vi "init_read_test.vi"() -> ()   [LabVIEW 2020, in "Avantes_bunch.lvclass"]
uses:
  Avantes_bunch.lvclass
  C:/dev/TRANCON/Classes/GeneralFunctionality/GeneralFunctionality.lvclass
  Config/config_names_def.ctl
  Config/Config.lvclass
  GeneralFunctionality/GeneralFunctionality.lvclass/GeneralFunctionality.ctl
  GeneralFunctionality/GeneralFunctionality.lvclass
panel:
  out "Waveform Graph 2":sgl[](graph)
  out "Waveform Graph":sgl[](graph)
  out "measuring":i32
  out "error out":errorcluster
  in  "Path":path=path "C:/Dev/TRANCON/settings/settingsDetector.ini"
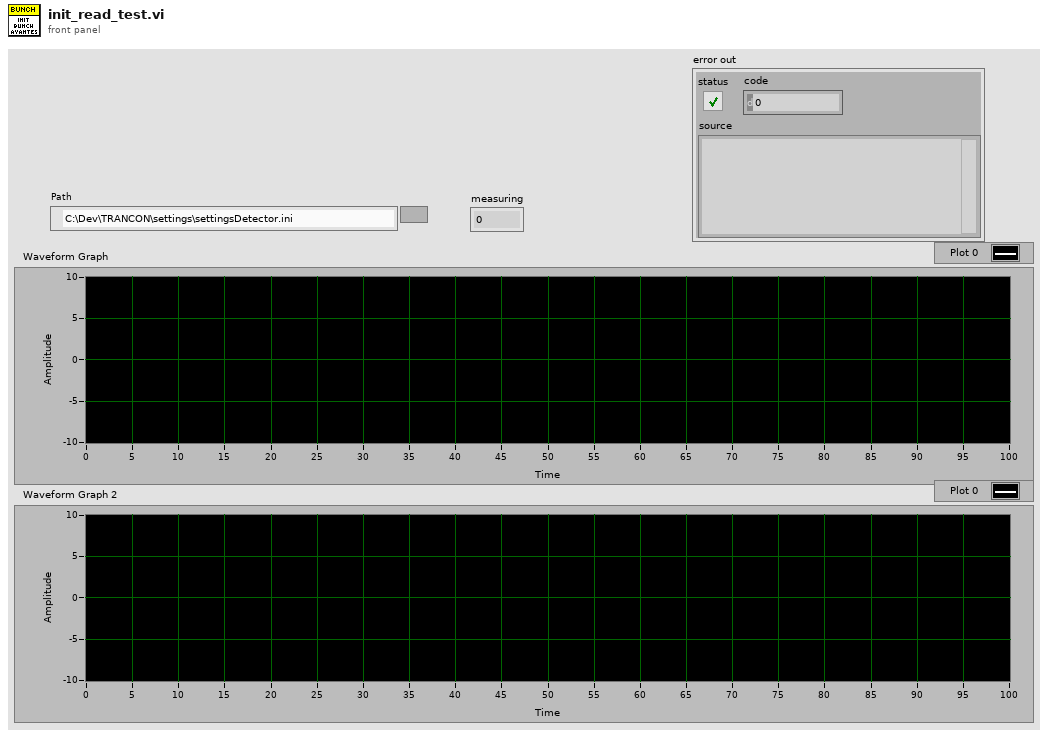
[diagram p1: front panel]
types:
  T1 = typedef "Config.lvclass/config_names_def.ctl" = string
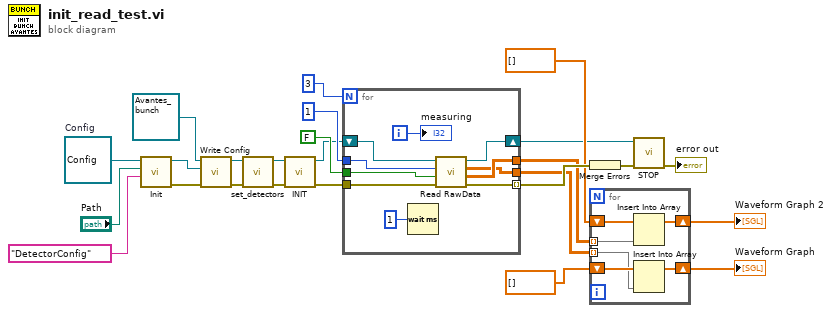
[diagram p0: block diagram]
diagram:
  w25 = refnum<class "Config.lvclass"> refnum  # Config
  n1 = call "Init.vi"("Name"=T1 "DetectorConfig" ("Config Name"), "Path"="Path", "Config in"=w25) -> ("error out"=w21:errorcluster, "Config out"=w20:refnum<class "Config.lvclass">)  [unwired: 7 in]
  n2 = call "Write Config.vi"("error in (no error)"=w21, "Config.lvclass"=w20, "GeneralFunctionality en entrée"=refnum<class "Avantes_bunch.lvclass"> refnum ("DET_BUNCH.lvclass")) -> ("error out"=w19:errorcluster, "GeneralFunctionality en sortie"=w18:refnum<class "Avantes_bunch.lvclass">)  [unwired: 7 in]
  n3 = call "set_detectors.vi"("error in (no error)"=w19, "DET_BUNCH in"=w18) -> ("error out"=w17:errorcluster, "DET_BUNCH out"=w16:refnum<class "Avantes_bunch.lvclass">)  [unwired: 8 in]
  n4 = call-dynamic "INIT.vi"("error in (no error)"=w17, "DET_BUNCH in"=w16) -> ("error out"=w14:errorcluster, "DET_BUNCH out"=w9:refnum<class "Avantes_bunch.lvclass">)  [unwired: 8 in]
  n5 = for {
    N: 3 -> [_]
    tunnel: w14 -> [w35]
    tunnel: [w34] -> w7
    tunnel: [w33] -> w8
    tunnel: 1 ("# of scans") -> [w32]
    tunnel: FALSE ("WCM_max_value") -> [w31]
    tunnel: [w29] -> w10 mode=indexing
    shift-right: [w28] -> w2
    shift-left: w9 -> [w27]
    i -> [w30]
    n6 = Wait (ms)(milliseconds to wait=u32 1) -> ()  [unwired: 1 out]
    n7 = call-dynamic "Read RawData.vi"("error in (no error)"=w35, "WCM_max_value"=w31, "# of scans"=w32, "DET_BUNCH in"=w27) -> ("error out"=w29:errorcluster, "Channel II"=w34:sgl[][], "Channel I"=w33:sgl[][], "DET_BUNCH out"=w28:refnum<class "Avantes_bunch.lvclass">)  [unwired: 3 in, 1 out]
    "measuring" <- w30
  }
  n8 = Merge Errors(w10) -> (w1:errorcluster)
  n9 = for {
    tunnel: w8 -> [w40] mode=indexing
    tunnel: w7 -> [w38] mode=indexing
    shift-right: [w39] -> w4
    shift-left: sgl[] [] ("Channel II") -> [w41]
    shift-right: [w36] -> w3
    shift-left: sgl[] [] ("Channel II") -> [w37]
    n10 = Insert Into Array(array=w37, new element=w38) -> (w36:sgl[])  [unwired: 1 in]
    n11 = Insert Into Array(array=w41, new element=w40) -> (w39:sgl[])  [unwired: 1 in]
  }
  "Waveform Graph" <- w4
  "Waveform Graph 2" <- w3
  n12 = call-dynamic "STOP.vi"("error in (no error)"=w1, "Stop in"=w2) -> ("error out"=→"error out":errorcluster)  [unwired: 8 in, 1 out]
